vi "Controller Mode.vi"(0 "VISA resource name":refnum<visa-resource-name>, 1 "Unit Address (1)":u8=1 min=1 max=254, 5 "Controller Mode (0: Auto)":u8(ring) items=["Auto", "Manual", "Off"], 11 "error in (no error)":errorcluster) -> (4 "VISA resource name out":refnum<visa-resource-name>, 15 "error out":errorcluster)   [LabVIEW 2010, in "Eurotherm 32xx Series.lvlib"]
doc: "This VI sets the controller mode to Auto, Manual or Off."
uses:
  <instrlib>/Eurotherm 32xx Series/Eurotherm 32xx Series.lvlib
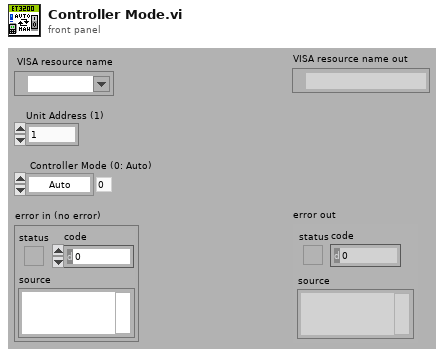
[diagram p1: front panel]
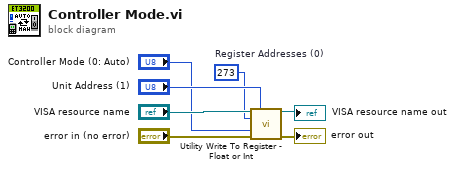
[diagram p0: block diagram]
diagram:
  w2 = u16 273  # Register Addresses (0)
  n1 = call <instrlib>:"Utility Write To Register - Float or Int.vi"("VISA resource name"="VISA resource name", "Unit Address (1)"="Unit Address (1)", "Register Address (0)"=w2, "Data (0)"="Controller Mode (0: Auto)", "error in (no error)"="error in (no error)") -> ("VISA resource name out"=→"VISA resource name out":refnum<visa-resource-name>, "error out"=→"error out":errorcluster)  [unwired: 9 in]
